vi "Initialize.vi"(7 "Reset (False)":bool, 8 "error in (no error)":errorcluster, 9 "Sample Rate (100 Hz)":u16=100 min=1 max=300 step=1, 11 "VISA resource name":refnum<visa-resource-name>) -> (0 "error out":errorcluster, 3 "VISA resource name out":refnum<visa-resource-name>)   [LabVIEW 2012, in "MicroStrain 3DM-GXx.lvlib"]
doc: "Establishes communication with the instrument. Call this VI before calling other instrument driver VIs for this instrument. You need to call the Initialize VI only once at the beginning of an application."
uses:
  <instrlib>/MicroStrain 3DM-GXx/MicroStrain 3DM-GXx.lvlib
panel:
  # "(c) 2009 - 2011 National Instruments.  ALL RIGHTS RESERVED."
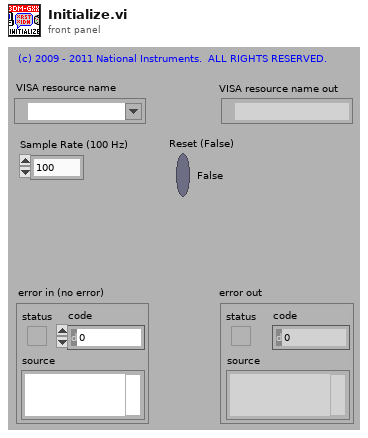
[diagram p1: front panel]
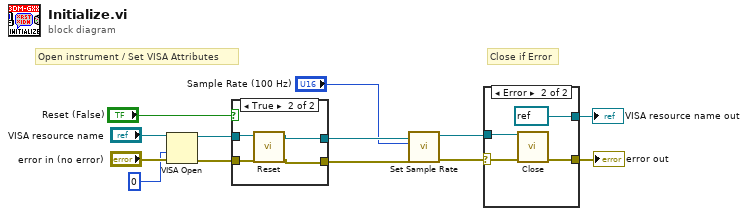
[diagram p0: block diagram]
diagram:
  # "Close if Error"
  # "Open instrument / Set VISA Attributes"
  n1 = VISA Open(access mode=u32 0, error in (no error)="error in (no error)", VISA resource name="VISA resource name") -> (VISA resource name=w5:refnum<visa-resource-name>, error out=w4:errorcluster)  [unwired: 2 in]
  n2 = case shown="True" "Reset (False)" {
    tunnel: w5 -> [w15 w19]
    tunnel: w4 -> [w14 w18]
    tunnel: [w15 w16] -> w3
    tunnel: [w14 w17] -> w2
    frame False {
    }
    frame True {
      n3 = call "Reset.vi"("error in (no error)"=w18, "VISA resource name"=w19) -> ("error out"=w17:errorcluster, "VISA resource name out"=w16:refnum<visa-resource-name>)  [unwired: 8 in]
    }
  }
  n4 = call <instrlib>:"Set Sample Rate.vi"("error in (no error)"=w2, "Sample Rate (100 Hz)"="Sample Rate (100 Hz)", "VISA resource name"=w3) -> ("error out"=w7:errorcluster, "VISA resource name out"=w8:refnum<visa-resource-name>)  [unwired: 7 in]
  n5 = case shown="Error" w7 {
    selector: w7 -> [w21 w22]
    tunnel: [w20 refnum<visa-resource-name> refnum ("VISA resource name out")] -> w10
    tunnel: [w21 w25] -> w9
    tunnel: w8 -> [w20 w23]
    frame No Error {
    }
    frame Error {
      n6 = call <instrlib>:"Close.vi"("error in (no error)"=w22, "VISA resource name"=w23) -> ("error out"=w25:errorcluster)  [unwired: 9 in]
    }
  }
  "VISA resource name out" <- w10
  "error out" <- w9
